vi "HapticSTM_raw.vi"() -> ()   [LabVIEW 2019]
uses:
  <vilib>/sound2/lvsound2.llb/Sampling Mode.ctl
  <vilib>/sound2/lvsound2.llb/Sound Data Format.ctl
  SubVIs/GlobalClicksHeight_raw.vi
  <vilib>/sound2/lvsound2.llb/Sound Output Set Volume (Single).vi
  <vilib>/sound2/lvsound2.llb/Sound Output Write (DBL Single).vi
  <vilib>/Utility/file.llb/Read Delimited Spreadsheet (DBL).vi
  <userlib>/HapticSTM/HapticSTM.lvlib
  <vilib>/ptbypt/NI_PtbyPt.lvlib
  <userlib>/Nanonis Prog Interface V5/Nanonis Prog Interface.lvlib
panel:
  in  "Version?":bool
  in  "Setpoint (pA)":dbl=100.0
  in  "Depth (pA)":dbl=280.0
  in  "Tab Control":T1(tab)
  out "ms/loop":u32=30
  in  "Z Write?":bool
  in  "Sound\nActivation":bool=TRUE
  in  "Sensitivity":dbl=1.0 format="%.1f"
  in  "Volume":dbl(slide)=50.0 scale=0.0..100.0
  in  "Device ID":u32
  out "function return":i32
  in  "Surface Shift (in)":dbl format="%.1f"
  in  "Scaling?":bool
  out "Setpoint (pA)":dbl
  in  "Maximum (pA)":dbl=7000.0
  out "Filtered Current (pA)":dbl format="%.1f"
  out "Current (pA)":dbl format="%.1f"
  out "Oy":dbl
  out "Ox":dbl
  out "W":dbl
  out "H":dbl
  out "Z Write":dbl format="%^.1e"
  out "Z Read":dbl format="%^#.1e"
  in  "Planing?":bool
  out "Button":bool
  out "Fy":dbl format="%.1f"
  out "Fz":dbl format="%.1f"
  out "Fx":dbl format="%.1f"
  out "x":dbl format="%.1f"
  out "y":dbl format="%.1f"
  out "z":dbl format="%0.1f"
  in  "Mode":u16(ring) items=["Log w/ Exp Z", "Log w/ Lin Z"]
  in  "Hardness":dbl=0.7 format="%.1f"
  in  "Reset Clicks":bool
  out "Clicks":i32
  in  "STOP":bool
  in  "START":bool
  out "Seq":i32
  out "SeqString":string
  out "Raw and Scaled Z Positions":T2(graph)
  out "Scaled Force and Current":T3(graph)
  # "Super Ultra Mega Haptic STM Controller 3000"
  # "Haptic Pen"
  # "Nanonis"
  # "Position"
  # "Force"
  # "Frame"
  # "Surface"
  # "Options"
  # "Addons"
  # "Test Data"
  # "Live"
  # "Sound Module"
  # "Small"
  # "Large"
  # "Current"
  # "Z Controller"
  # "No"
  # "Yes"
  # "Planing"
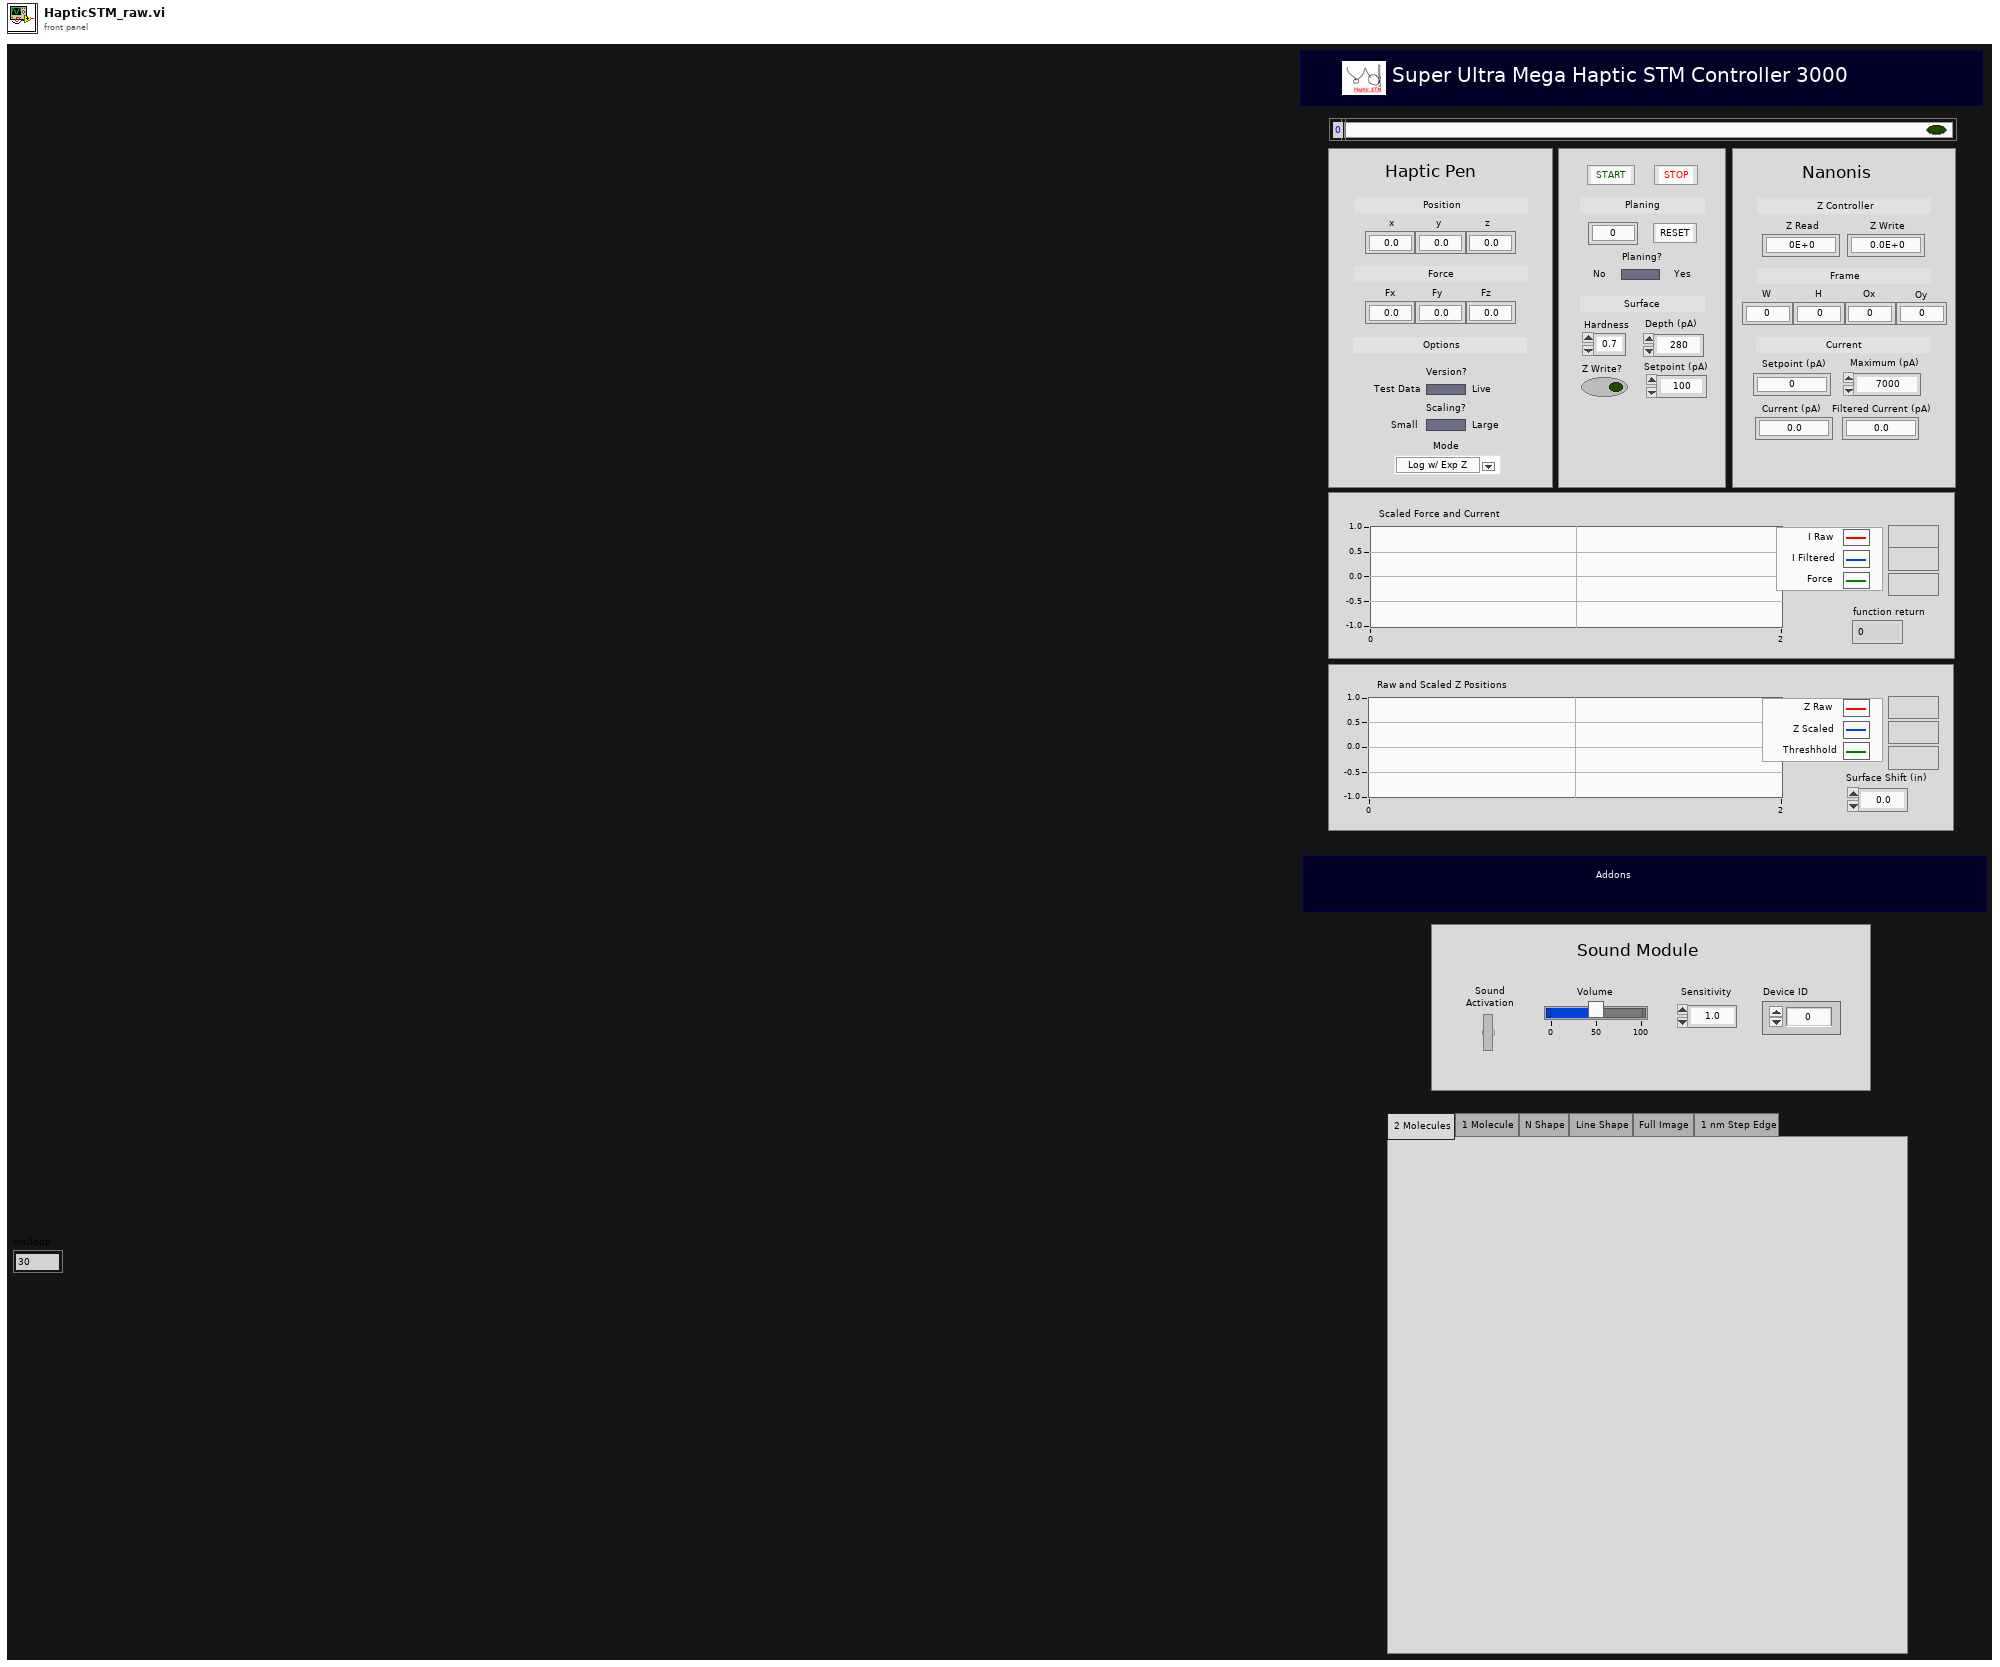
[diagram p1: front panel]
types:
  T1 = enum32{"2 Molecules", "1 Molecule", "N Shape", "Line Shape", "Full Image", "1 nm Step Edge"}
  T2 = cluster{dbl, "function return":dbl, "function return":dbl}
  T3 = cluster{"Current (pA)":dbl, "Filtered Current (pA)":dbl, dbl}
  T4 = typedef "Sound Data Format.ctl" = cluster{"sample rate (S/s)":dbl, "number of channels":i32, "bits per sample":i32}
  T5 = typedef "Sampling Mode.ctl" = i32
  T6 = cluster{"Size (m)":cluster{"Width":sgl, "Height":sgl}, "Center coordinates (m)":cluster{"Xc":sgl, "Yc":sgl}}
  T7 = typedef "Sound Output Task ID.ctl" = u32
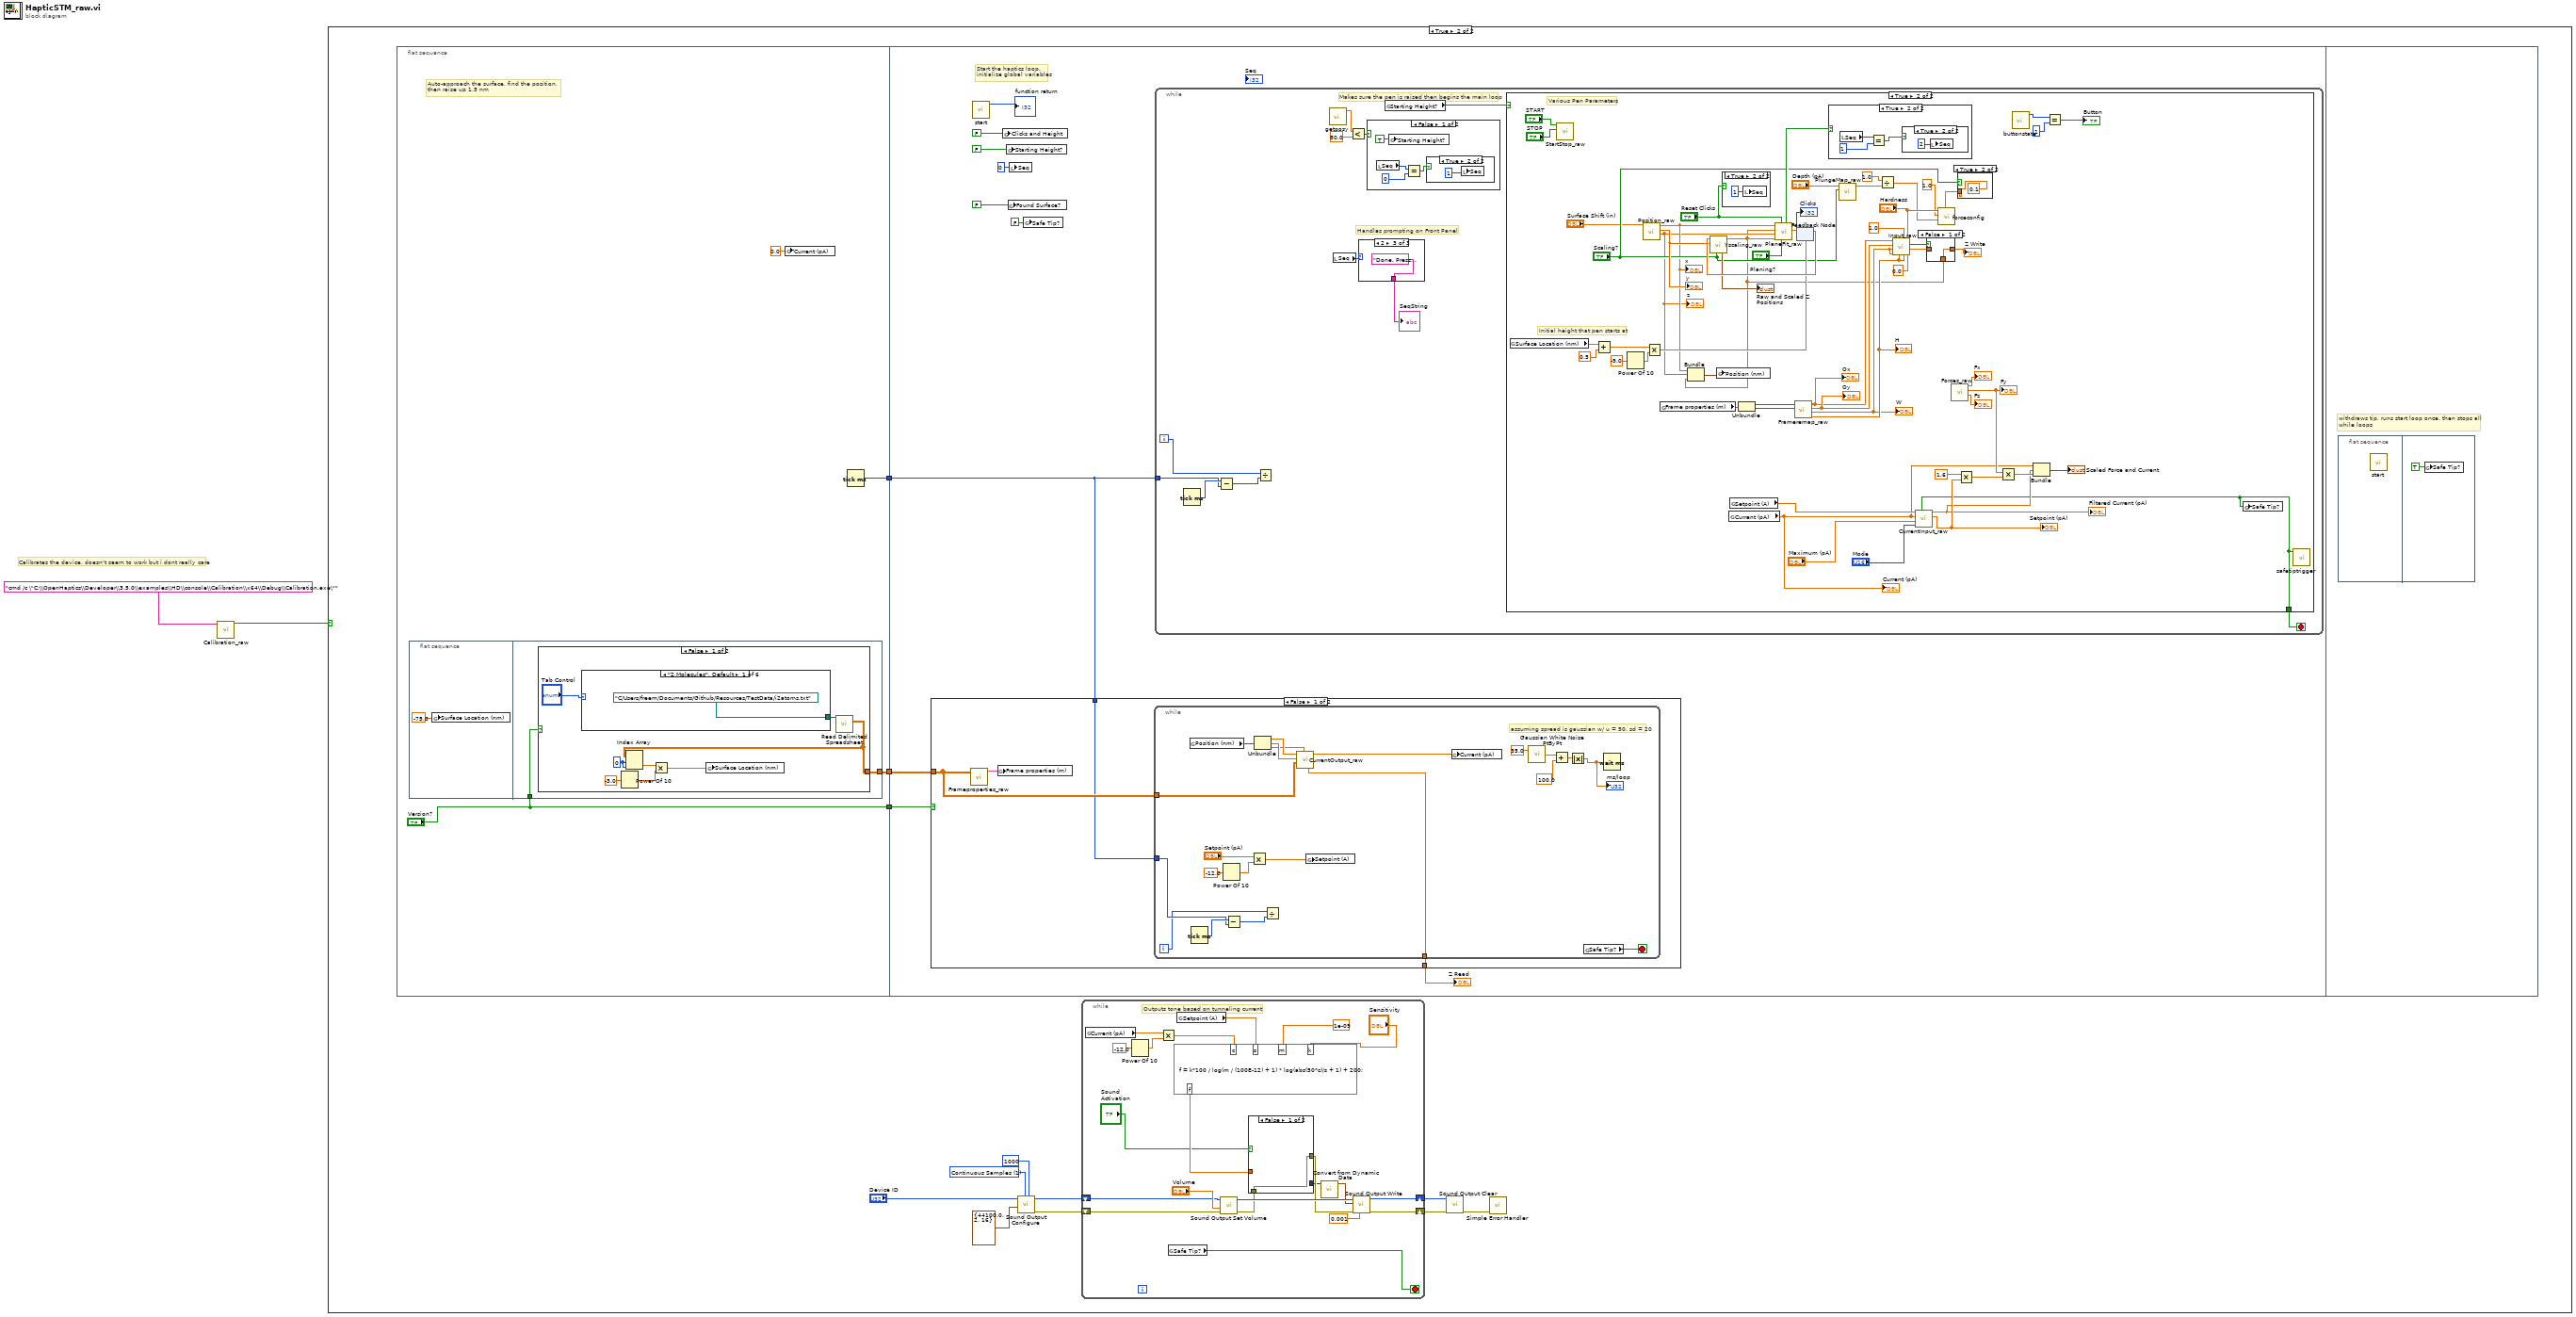
[diagram p0: block diagram]
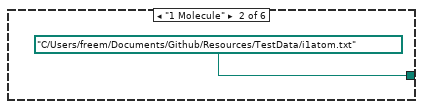
[diagram p3: hidden frame]
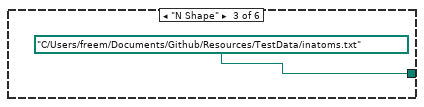
[diagram p4: hidden frame]
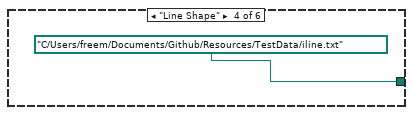
[diagram p5: hidden frame]
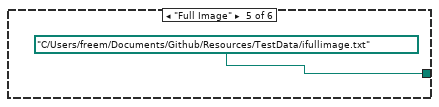
[diagram p6: hidden frame]
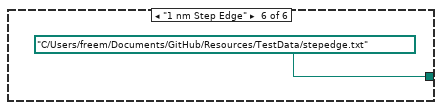
[diagram p7: hidden frame]
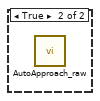
[diagram p8: hidden frame]
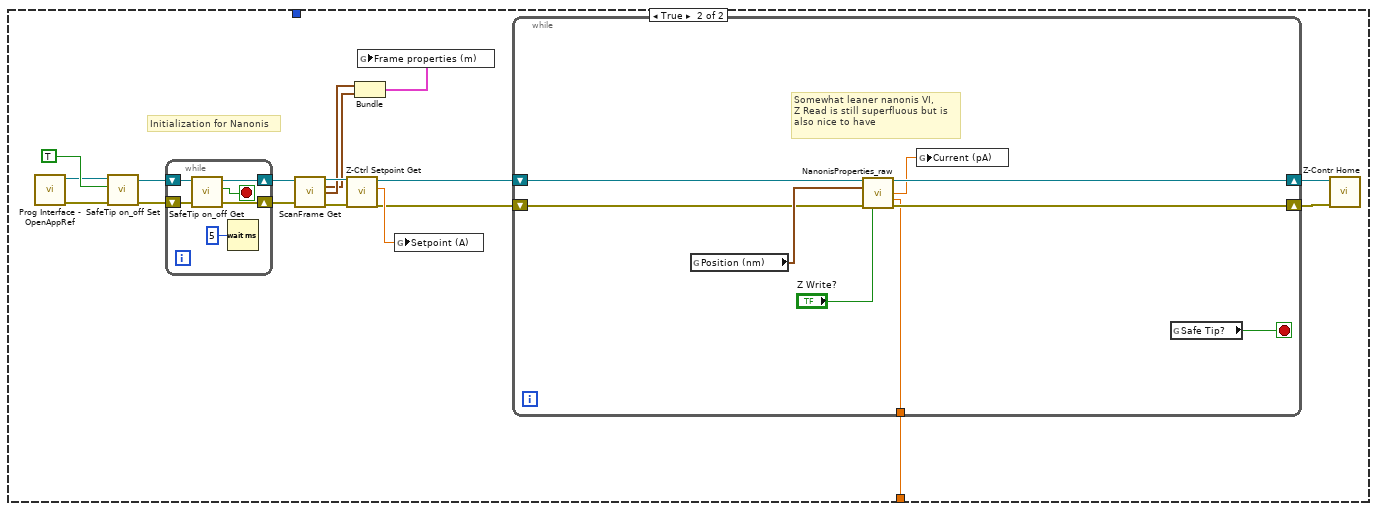
[diagram p9: hidden frame]
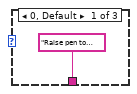
[diagram p10: hidden frame]
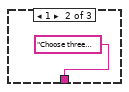
[diagram p11: hidden frame]
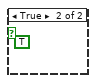
[diagram p13: hidden frame]
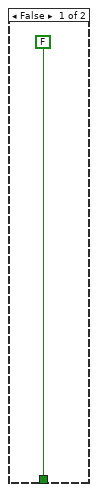
[diagram p14: hidden frame]
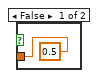
[diagram p15: hidden frame]
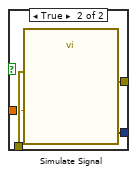
[diagram p20: hidden frame]
diagram:
  # "Calibrates the device, doesn't seem to work but i dont really care"
  n1 = call "Calibration_raw.vi"("command line"="cmd /c \"C:\\OpenHaptics\\Developer\\3.5.0\\examples\\HD\\console\\Calibration\\x64\\Debug\\Calibration.exe\"") -> ("Calibration Complete?"=w2:bool)  [unwired: 10 in]
  n2 = case shown="True" w2 {
    frame False {
    }
    frame True {
      w13 = T5 1 items=["Finite Samples", "Continuous Samples"] ("sample mode")
      n3 = flat-sequence {
        tunnel: ["Version?"] -> w5
        tunnel: [w17] -> w4
        tunnel: [w16] -> w3
        tunnel: w5 -> [w38]
        tunnel: w4 -> [w37]
        tunnel: w3 -> [w36]
        frame #0 {
          # "Auto-approach the surface, find the position, \nthen raise up 1.5 nm"
          n4 = flat-sequence {
            tunnel: "Version?" -> [w21]
            tunnel: [w20] -> w17
            frame #0 {
              n5 = global write "GlobalClicksHeight_raw.vi" "Surface Location (nm)"(-75.0 ("Surface Location")) -> ()
            }
            frame #1 {
              n6 = case shown="False" w21 {
                tunnel: [w27 _] -> w20
                frame False {
                  w26 = 0 ("index (row)")
                  n7 = case shown="\"2 Molecules\", Default" "Tab Control" {
                    tunnel: [path "C:/Users/freem/Documents/Github/Resources/TestData/i2atoms.txt" ("file path (dialog if empty)") path "C:/Users/freem/Documents/Github/Resources/TestData/i1atom.txt" ("file path (dialog if empty)") path "C:/Users/freem/Documents/Github/Resources/TestData/inatoms.txt" ("file path (dialog if empty)") path "C:/Users/freem/Documents/Github/Resources/TestData/iline.txt" ("file path (dialog if empty)") path "C:/Users/freem/Documents/Github/Resources/TestData/ifullimage.txt" ("file path (dialog if empty)") path "C:/Users/freem/Documents/GitHub/Resources/TestData/stepedge.txt" ("file path (dialog if empty)")] -> w29
                    frame "2 Molecules", Default {
                    }
                    frame "1 Molecule" {
                    }
                    frame "N Shape" {
                    }
                    frame "Line Shape" {
                    }
                    frame "Full Image" {
                    }
                    frame "1 nm Step Edge" {
                    }
                  }
                  n8 = Power Of 10(x=-3.0) -> (10^x=w24:dbl)
                  n9 = call-poly <vilib>:"Read Delimited Spreadsheet.vi"("file path (dialog if empty)"=w29) -> ("all rows"=w27:dbl[][])  [unwired: 9 in, 5 out]
                  n10 = Index Array(array=w27, index (row)=w26, index (col)=w26) -> (element=w25:dbl)
                  n11 = Multiply(x=w25, y=w24) -> (x*y=w22:dbl)
                  n12 = global write "GlobalClicksHeight_raw.vi" "Surface Location (nm)"(w22) -> ()
                }
                frame True {
                  n13 = call "AutoApproach_raw.vi"() -> ()  [unwired: 12 in]
                }
              }
            }
          }
          n14 = global write "GlobalClicksHeight_raw.vi" "Current (pA)"(0.0 ("Current (pA)")) -> ()
          n15 = Tick Count (ms)() -> (millisecond timer value=w16:u32)
        }
        frame #1 {
          # "Start the haptics loop,\ninitialize global variables"
          n16 = case shown="False" w38 {
            tunnel: [w49 w74] -> w39
            tunnel: w37 -> [w48 _]
            tunnel: w36 -> [w46 _]
            frame False {
              n17 = call "Frameproperties_raw.vi"("array"=w48) -> ("Frame properties"=w47:cluster{cluster{dbl, dbl}, cluster{dbl, dbl}})  [unwired: 10 in]
              n18 = global write "GlobalClicksHeight_raw.vi" "Frame properties (m)"(w47) -> ()
              n19 = while {
                tunnel: [w56] -> w49
                tunnel: w48 -> [w55]
                tunnel: w46 -> [w58]
                i -> [w57]
                stop <- w52 stop-if-true
                # "assuming spread is gaussian w/ u = 50, sd = 20"
                n20 = global read "GlobalClicksHeight_raw.vi" "Position (nm)"() -> (w65:cluster{"X":dbl, "Z":dbl, "Y":dbl})
                n21 = Tick Count (ms)() -> (millisecond timer value=w59:u32)
                n22 = Power Of 10(x=-12.0) -> (10^x=w63:dbl)
                n23 = Subtract(x=w59, y=w58) -> (x-y=w60:u32)
                n24 = Multiply(x="Setpoint (pA)", y=w63) -> (x*y=w61:dbl)
                n25 = Unbundle(w65) -> ("X"=w53:dbl, "Z"=w54:dbl, "Y"=w50:dbl)
                n26 = Divide(x=w57, y=w60) -> ()  [unwired: 1 out]
                n27 = call "CurrentOutput_raw.vi"("y scaled"=w50, "array"=w55, "Z Input"=w54, "X Input"=w53) -> ("Current Out (pA)"=w51:dbl, "Zread"=w56:dbl)  [unwired: 3 in, 3 out]
                n28 = global write "GlobalClicksHeight_raw.vi" "Setpoint (A)"(w61) -> ()
                n29 = global write "GlobalClicksHeight_raw.vi" "Current (pA)"(w51) -> ()
                n30 = call <vilib>:"Gaussian White Noise PtByPt.vi"("standard deviation"=35.0) -> ("Gaussian white noise"=w69:dbl)  [unwired: 2 in]
                n31 = Add(x=w69, y=100.0) -> (x+y=w67:dbl)
                n32 = Absolute Value(x=w67) -> (abs(x)=w66:dbl)
                "ms/loop" <- w66
                n33 = global read "GlobalClicksHeight_raw.vi" "Safe Tip?"() -> (w52:bool)
                n34 = Wait (ms)(milliseconds to wait=w66) -> ()  [unwired: 1 out]
              }
            }
            frame True {
              # "Initialization for Nanonis"
              n35 = call <userlib>:"Prog Interface - OpenAppRef.vi"() -> ("Error out"=w86:errorcluster, "Application reference"=w87:refnum<vi>)  [unwired: 6 in]
              n36 = call <userlib>:"SafeTip on_off Set.vi"("error in (no error)"=w86, "SafeTip ON/OFF"=TRUE, "Application ref in"=w87) -> ("error out"=w84:errorcluster, "Application ref out"=w85:refnum<vi>)  [unwired: 7 in]
              n37 = while {
                shift-right: [w91] -> w83
                shift-left: w85 -> [w93]
                shift-right: [w90] -> w82
                shift-left: w84 -> [w92]
                stop <- w94 stop-if-true
                n38 = call <userlib>:"SafeTip on_off Get.vi"("error in (no error)"=w92, "Application ref in"=w93) -> ("error out"=w90:errorcluster, "SafeTip on/off status"=w94:bool, "Application ref out"=w91:refnum<vi>)  [unwired: 7 in]
                n39 = Wait (ms)(milliseconds to wait=u32 5) -> ()  [unwired: 1 out]
              }
              n40 = call <userlib>:"ScanFrame Get.vi"("Application ref in"=w83, "error in (no error)"=w82) -> ("Application ref out"=w81:refnum<vi>, "Center coordinates (m)"=w71:cluster{"Xc":sgl, "Yc":sgl}, "Size (m)"=w72:cluster{"Width":sgl, "Height":sgl}, "error out"=w80:errorcluster)  [unwired: 9 in, 1 out]
              n41 = call <userlib>:"Z-Ctrl Setpoint Get.vi"("error in (no error)"=w80, "Application ref in"=w81) -> ("error out"=w77:errorcluster, "Z Controller setpoint"=w79:sgl, "Application ref out"=w78:refnum<vi>)  [unwired: 6 in]
              n42 = Bundle("Size (m)"=w72, "Center coordinates (m)"=w71) -> (w73:T6)  [unwired: 1 in]
              n43 = global write "GlobalClicksHeight_raw.vi" "Frame properties (m)"(w73) -> ()
              n44 = global write "GlobalClicksHeight_raw.vi" "Setpoint (A)"(w79) -> ()
              n45 = while {
                shift-right: [w97] -> w75
                shift-left: w77 -> [w99]
                shift-right: [w98] -> w76
                shift-left: w78 -> [w101]
                tunnel: [w95] -> w74
                stop <- w103 stop-if-true
                # "Somewhat leaner nanonis VI, \nZ Read is still superfluous but is\nalso nice to have"
                n46 = global read "GlobalClicksHeight_raw.vi" "Position (nm)"() -> (w102:cluster{"X":dbl, "Z":dbl, "Y":dbl})
                n47 = call "NanonisProperties_raw.vi"("Application ref in"=w101, "Position (nm)"=w102, "error in (no error)"=w99, "Z Write?"="Z Write?") -> ("Application ref out"=w98:refnum<vi>, "Current (pA)"=w96:sgl, "Z Read (m)"=w95:sgl, "error out"=w97:errorcluster)  [unwired: 8 in]
                n48 = global write "GlobalClicksHeight_raw.vi" "Current (pA)"(w96) -> ()
                n49 = global read "GlobalClicksHeight_raw.vi" "Safe Tip?"() -> (w103:bool)
              }
              n50 = call <userlib>:"Z-Contr Home.vi"("Error in (no error)"=w75, "Application ref in"=w76) -> ()  [unwired: 8 in, 2 out]
            }
          }
          "Z Read" <- w39
          n51 = call <userlib>:"start.vi"() -> ("function return"=→"function return":i32)  [unwired: 11 in]
          n52 = global write "GlobalClicksHeight_raw.vi" "Clicks and Height"(FALSE ("Clicks and Height")) -> ()
          n53 = global write "GlobalClicksHeight_raw.vi" "Starting Height?"(FALSE ("Clicks and Height")) -> ()
          n54 = global write "GlobalClicksHeight_raw.vi" "Found Surface?"(FALSE ("Clicks and Height")) -> ()
          n55 = local write "Seq"(0 ("Seq")) -> ()
          n56 = global write "GlobalClicksHeight_raw.vi" "Safe Tip?"(FALSE ("Safe Tip?")) -> ()
          n57 = while {
            tunnel: w36 -> [w104]
            i -> [w107]
            stop <- w108 stop-if-true
            # "Makes sure the pen is raised then begins the main loop"
            # "Handles prompting on Front Panel"
            n58 = Tick Count (ms)() -> (millisecond timer value=w105:u32)
            n59 = Subtract(x=w105, y=w104) -> (x-y=w106:u32)
            n60 = Divide(x=w107, y=w106) -> ()  [unwired: 1 out]
            n61 = call <userlib>:"getposy.vi"() -> ("function return"=w114:dbl)  [unwired: 11 in]
            n62 = local read "Seq"() -> (w110:i32)
            n63 = Less?(x=w114, y=80.0) -> (x < y?=w112:bool)
            n64 = case shown="2" w110 {
              tunnel: ["Raise pen to begin." "Choose three points, then raise the arm to plane." "Done. Press 'STOP' to stop at anytime."] -> w109
              frame 0, Default {
              }
              frame 1 {
              }
              frame 2 {
              }
            }
            "SeqString" <- w109
            n65 = case shown="False" w112 {
              frame False {
                n66 = local read "Seq"() -> (w120:i32)
                n67 = global write "GlobalClicksHeight_raw.vi" "Starting Height?"(TRUE ("Starting Height?")) -> ()
                n68 = Equal?(x=w120, y=0) -> (x = y?=w118:bool)
                n69 = case shown="True" w118 {
                  frame False {
                  }
                  frame True {
                    n70 = local write "Seq"(1 ("Seq")) -> ()
                  }
                }
              }
              frame True {
                (unwired) TRUE ("Clicks and Height")
              }
            }
            n71 = global read "GlobalClicksHeight_raw.vi" "Starting Height?"() -> (w111:bool)
            n72 = case shown="True" w111 {
              tunnel: [FALSE ("Current Maxed?") w128] -> w108
              frame False {
              }
              frame True {
                # "Initial height that pen starts at"
                # "Various Pen Parameters"
                n73 = global read "GlobalClicksHeight_raw.vi" "Surface Location (nm)"() -> (w143:dbl)
                n74 = call "StartStop_raw.vi"("STOP"="STOP", "START"="START") -> ()  [unwired: 10 in]
                n75 = Add(x=w143, y=0.5) -> (x+y=w140:dbl)
                n76 = Power Of 10(x=-9.0) -> (10^x=w139:dbl)
                n77 = call "Position_raw.vi"("Shift"="Surface Shift (in)") -> ("Z"=w131:dbl, "Y"=w169:dbl, "X"=w132:dbl)  [unwired: 8 in]
                "x" <- w132
                "y" <- w169
                "z" <- w131
                n78 = Multiply(x=w140, y=w139) -> (x*y=w141:dbl)
                n79 = global read "GlobalClicksHeight_raw.vi" "Frame properties (m)"() -> (w127:cluster{cluster{dbl, dbl}, cluster{dbl, dbl}})
                n80 = case shown="True" "Reset Clicks" {
                  frame False {
                  }
                  frame True {
                    n81 = local write "Seq"(1 ("Seq")) -> ()
                  }
                }
                n82 = global read "GlobalClicksHeight_raw.vi" "Current (pA)"() -> (w124:dbl)
                "Current (pA)" <- w124
                n83 = global read "GlobalClicksHeight_raw.vi" "Setpoint (A)"() -> (w129:dbl)
                n84 = Unbundle(w127) -> (w126:cluster{dbl, dbl}, w125:cluster{dbl, dbl})
                n85 = call "Frameremap_raw.vi"("Frame Origin (m)"=w125, "Frame Size (m)"=w126) -> ("FH (nm)"=w153:dbl, "FW (nm)"=w152:dbl, "Z Origin (nm)"=w151:dbl, "X Origin (nm)"=w150:dbl)  [unwired: 6 in]
                "H" <- w153
                "W" <- w152
                "Ox" <- w150
                "Oy" <- w151
                n86 = feedback #1(w141) -> (w175:dbl)
                n87 = call "Yscaling_raw.vi"("Scaling?"="Scaling?", "Y"=w169, "Plane Height (m)"=w175) -> ("y scaled (m)"=w130:dbl, "Zpos Graph (nm)"=→"Raw and Scaled Z Positions":T2)  [unwired: 7 in]
                n88 = Bundle("X"=w132, "Z"=w131, "y scaled (m)"=w130) -> (w133:cluster{"X":dbl, "Z":dbl, "y scaled (m)":dbl})  [unwired: 1 in]
                n89 = global write "GlobalClicksHeight_raw.vi" "Position (nm)"(w133) -> ()
                n90 = call "PlaneFit_raw.vi"("Planing y/n?"="Planing?", "Reset Clicks"="Reset Clicks", "Y PEN"=w130, "Z"=w131, "Nano Z"=w130, "X"=w132) -> ("Plane Height (m)"=w176:dbl, "Clicks"=→"Clicks":i32, "Planing Done?"=w162:bool)  [unwired: 3 in]
                n91 = feedback-in #1(w176) -> ()
                n92 = case shown="True" w162 {
                  frame False {
                  }
                  frame True {
                    n93 = local read "Seq"() -> (w189:i32)
                    n94 = Equal?(x=w189, y=1) -> (x = y?=w187:bool)
                    n95 = case shown="True" w187 {
                      frame False {
                      }
                      frame True {
                        n96 = local write "Seq"(2 ("Seq")) -> ()
                      }
                    }
                  }
                }
                n97 = call "PlungeMap_raw.vi"("Scaling?"="Scaling?", "Input (pA)"="Depth (pA)") -> ("output"=w144:dbl)  [unwired: 9 in]
                n98 = Divide(x=1.0, y=w144) -> (x/y=w154:dbl)
                n99 = call "Input_raw.vi"("Current * 10^input"=0.0, "Sensitivity"="Hardness", "Scopez"=w153, "Drag"=1.0, "FH"=w153, "FW"=w152, "Scopex"=w152, "Z origin"=w151, "X origin"=w150) -> ("Scaled Current"=w156:dbl, "feedback"=w158:bool)  [unwired: 1 in]
                n100 = call "CurrentInput_raw.vi"("Mode"="Mode", "Maximum (pA)"="Maximum (pA)", "Current (pA)"=w124, "Setpoint (A)"=w129) -> ("Setpoint (pA)"=w146:dbl, "Filtered Current (pA)"=w137:dbl, "Safetip?"=w128:bool)  [unwired: 5 in]
                "Filtered Current (pA)" <- w137
                "Setpoint (pA)" <- w146
                n101 = case shown="False" w158 {
                  tunnel: [w184 w185] -> w157
                  tunnel: w156 -> [_ w185]
                  tunnel: w130 -> [w184 _]
                  frame False {
                  }
                  frame True {
                  }
                }
                "Z Write" <- w157
                n102 = call "Forces_raw.vi"() -> ("Fz"=→"Fz":dbl, "Fy"=w173:dbl, "Fx"=→"Fx":dbl)  [unwired: 9 in]
                "Fy" <- w173
                n103 = case shown="True" "Scaling?" {
                  tunnel: [0.5 0.1] -> w136
                  frame False {
                  }
                  frame True {
                  }
                }
                n104 = call <userlib>:"forceconfig.vi"("spc"=w136, "c"=w154, "b"=1.0, "a"="Hardness") -> ()  [unwired: 8 in]
                n105 = Multiply(x=1.6 ("y"), y=w146) -> (x*y=w170:dbl)
                n106 = Multiply(x=w173, y=w170) -> (x*y=w172:dbl)
                n107 = call <userlib>:"buttonstate.vi"() -> ("function return"=w168:i32)  [unwired: 11 in]
                n108 = Bundle("Current (pA)"=w124, "Filtered Current (pA)"=w137, w172) -> (→"Scaled Force and Current":T3)  [unwired: 1 in]
                n109 = Equal?(x=w168, y=1) -> (x = y?=→"Button":bool)
                n110 = global write "GlobalClicksHeight_raw.vi" "Safe Tip?"(w128) -> ()
                n111 = call <userlib>:"safetiptrigger.vi"("triggered"=w128) -> ()  [unwired: 11 in]
              }
            }
          }
        }
        frame #2 {
          # "withdraws tip, runs start loop once, then stops all\nwhile loops"
          n112 = flat-sequence {
            frame #0 {
              n113 = call <userlib>:"start.vi"() -> ()  [unwired: 11 in, 1 out]
            }
            frame #1 {
              n114 = global write "GlobalClicksHeight_raw.vi" "Safe Tip?"(TRUE ("Safe Tip?")) -> ()
            }
          }
        }
      }
      n115 = call <vilib>:"Sound Output Configure.vi"("number of samples/ch"=1000 ("Number of Samples/ch"), "sample mode"=w13, "sound format"=T4 {"sample rate (S/s)"=44100.0, "number of channels"=2, "bits per sample"=16} ("Sound Format"), "device ID"="Device ID") -> ("error out"=w9:errorcluster, "task ID"=w10:T7)  [unwired: 6 in]
      n116 = while {
        shift-right: [w204] -> w8
        shift-left: w10 -> [w206]
        shift-right: [w203] -> w7
        shift-left: w9 -> [w205]
        stop <- w193 stop-if-true
        # "Outputs tone based on tunneling current"
        n117 = global read "GlobalClicksHeight_raw.vi" "Current (pA)"() -> (w196:dbl)
        n118 = Power Of 10(x=-12.0) -> (10^x=w198:dbl)
        n119 = Multiply(x=w196, y=w198) -> (x*y=w195:dbl)
        n120 = global read "GlobalClicksHeight_raw.vi" "Safe Tip?"() -> (w193:bool)
        n121 = global read "GlobalClicksHeight_raw.vi" "Setpoint (A)"() -> (w200:dbl)
        n122 = formula code="f = k*100 / log(m / (100E-12) + 1) * log(abs(50*c)/s + 1) + 200;"("c"=w195, "m"=1e-09 ("input variable"), "s"=w200, "k"="Sensitivity") -> ("f"=w199:dbl)
        n123 = call-poly <vilib>:"Sound Output Set Volume.vi"("error in (no error)"=w205, "volume"="Volume", "task ID"=w206) -> ("error out"=w209:errorcluster, "task ID out"=w212:T7)  [unwired: 7 in]
        n124 = case shown="False" "Sound\nActivation" {
          tunnel: w209 -> [w213 w217]
          tunnel: [w213 w216] -> w208
          tunnel: [_ w215] -> w207
          tunnel: w199 -> [_ w214]
          frame False {
          }
          frame True {
            n125 = call "Simulate Signal"("Frequency"=w214, "error in (no error)"=w217) -> ("Sine"=w215:dynamicdata, "error out"=w216:errorcluster)  [unwired: 12 in]
          }
        }
        n126 = call "Convert from Dynamic Data"("Dynamic Data Type"=w207) -> ("Waveform"=w210:waveform(dbl))  [unwired: 3 in]
        n127 = call-poly <vilib>:"Sound Output Write.vi"("timeout (sec)"=0.001, "error in (no error)"=w208, "data"=w210, "task ID"=w212) -> ("error out"=w203:errorcluster, "task ID out"=w204:T7)  [unwired: 6 in]
      }
      n128 = call <vilib>:"Sound Output Clear.vi"("error in (no error)"=w7, "task ID"=w8) -> ("error out"=w12:errorcluster)  [unwired: 9 in]
      n129 = call <vilib>:"Simple Error Handler.vi"("error in (no error)"=w12) -> ()  [unwired: 4 in, 5 out]
    }
  }
